vi "Update Outputs.vi"() -> ()   [LabVIEW 2012]
uses:
  <vilib>/Rock Robotics/WPI/Solenoid/WPI_SolenoidValue.ctl
  <vilib>/Rock Robotics/WPI/RobotDrive/WPI_RobotDriveGetSetRefNum.vi
  Robot Global Data.vi
  <vilib>/Rock Robotics/WPI/Solenoid/WPI_SolenoidSetEnum.vi
  <vilib>/Rock Robotics/WPI/RobotDrive/WPI_RobotDriveArcadeDrive_Standard(NoSaturation).vi
panel:
  out "Gyro Angle":dbl(knob) scale=0.0..360.0
  out "Loop Time 2":u32(graph)
  out "Right Distance (ft)":dbl
  out "Left Distance (ft)":dbl
  out "Right Rate":dbl(graph)
  out "Left Rate":dbl(graph)
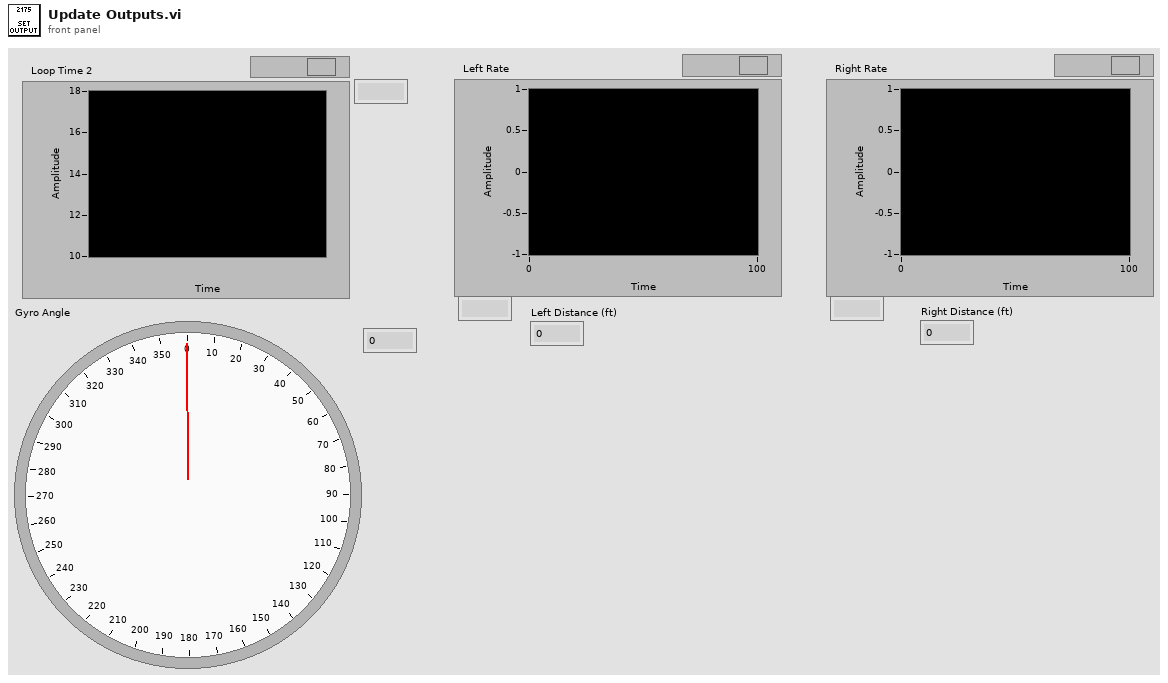
[diagram p1: front panel]
types:
  T1 = typedef "WPI_SolenoidDevRef.ctl" = cluster{"DevStatus":errorcluster, "Solenoid Module":T2, "Forward Solenoid Channel":T3, "Reverse Solenoid Channel":T3}
  T2 = typedef "FPGA_TypedefSolenoidModule.ctl" = enum16{"Solenoid Module 1", "Solenoid Module 2"}
  T3 = typedef "WPI_SolenoidChannel.ctl" = enum8{"Solenoid 1", "Solenoid 2", "Solenoid 3", "Solenoid 4", "Solenoid 5", "Solenoid 6", "Solenoid 7", "Solenoid 8", "Invalid"}
  T4 = typedef "WPI_RobotDriveDevRef.ctl" = cluster{"DevStatus":errorcluster, "Motors[]":T5[], "Square Inputs":bool, "Max Output":dbl, "Isochronous":bool}
  T5 = typedef "WPI_MotorControlDeviceRef.ctl" = cluster{"DeviceStatus":errorcluster, "Type":enum16{"PWM", "CAN"}, "PWM":cluster{"Digital Module":T6, "PWM Channel":T7, "DeadBand":T8}, "CAN":cluster{"Device Number":u8, "Control Mode":T9, "Semaphore":T10, "Max Vout":dbl}, "Invert":bool, "TransformRef":T11, "InvTransformRef":T11}
  T6 = typedef "FPGA_TypedefDigitalModule.ctl" = enum16{"Digital Module 1", "Digital Module 2"}
  T7 = typedef "FPGA_DIOPWMChannel.ctl" = enum8{"PWM 1", "PWM 2", "PWM 3", "PWM 4", "PWM 5", "PWM 6", "PWM 7", "PWM 8", "PWM 9", "PWM 10", "Invalid"}
  T8 = typedef "WPI_PWMDeadband.ctl" = cluster{"Name":string, "maxPositivePwm":i32, "minPositivePwm":i32, "centerPwm":i32, "maxNegativePwm":i32, "minNegativePwm":i32, "angularRange":u16}
  T9 = typedef "WPI_CANJaguar_ControlMode.ctl" = enum8{"Percent VBus", "Current", "Speed", "Position", "Voltage"}
  T10 = typedef "Semaphore RefNum" = refnum<k1>
  T11 = typedef "WPI_PWMTransform_ConPane.ctl" = refnum<vi>
  T12 = typedef "WPI_DigitalInputDevRef.ctl" = cluster{"DevStatus":errorcluster, "DIO Channel":T13, "Digital Module":T6}
  T13 = typedef "FPGA_DIOChannel.ctl" = enum8{"DIO 1", "DIO 2", "DIO 3", "DIO 4", "DIO 5", "DIO 6", "DIO 7", "DIO 8", "DIO 9", "DIO 10", "DIO 11", "DIO 12", "DIO 13", "DIO 14", "Invalid"}
  T14 = typedef "WPI_EncoderDevRef.ctl" = cluster{"DevStatus":errorcluster, "EncoderIndex":T15, "CounterIndex":T16, "DistancePerCount":dbl, "Decoding Type":T17}
  T15 = typedef "FPGA_EncoderIdx.ctl" = enum8{"Enc 0", "Enc 1", "Enc 2", "Enc 3", "Invalid"}
  T16 = typedef "FPGA_CounterCtrSystemIndex.ctl" = enum8{"Ctr 0", "Ctr 1", "Ctr 2", "Ctr 3", "Ctr 4", "Ctr 5", "Ctr 6", "Ctr 7", "Invalid"}
  T17 = typedef "WPI_EncoderType.ctl" = enum16{"1x", "2x", "4x"}
  T18 = typedef "WPI_SolenoidValue.ctl" = enum16{"Off", "On", "Forward", "Reverse"}
  T19 = typedef "WPI_GyroDevRef.ctl" = cluster{"DevStatus":errorcluster, "Analog Module":T20, "Analog Channel":T21, "Offset":dbl, "Gain (VoltsPerDegree/Second)":dbl}
  T20 = typedef "FPGA_TypedefAnalogModule.ctl" = enum16{"Analog Module 1", "Analog Module 2"}
  T21 = typedef "FPGA_AIChannel.ctl" = enum8{"AI 1", "AI 2", "AI 3", "AI 4", "AI 5", "AI 6", "AI 7", "AI 8", "Invalid"}
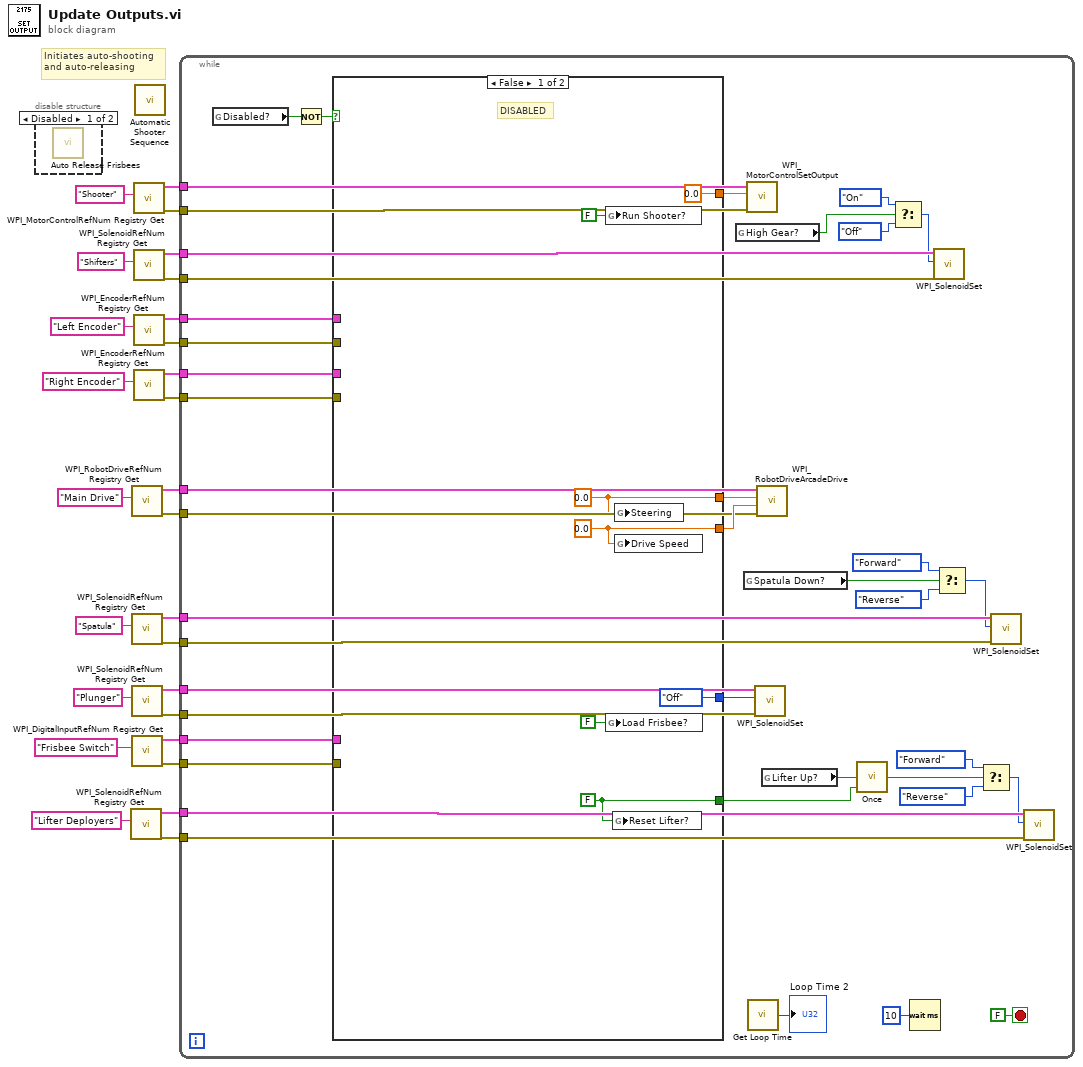
[diagram p0: block diagram]
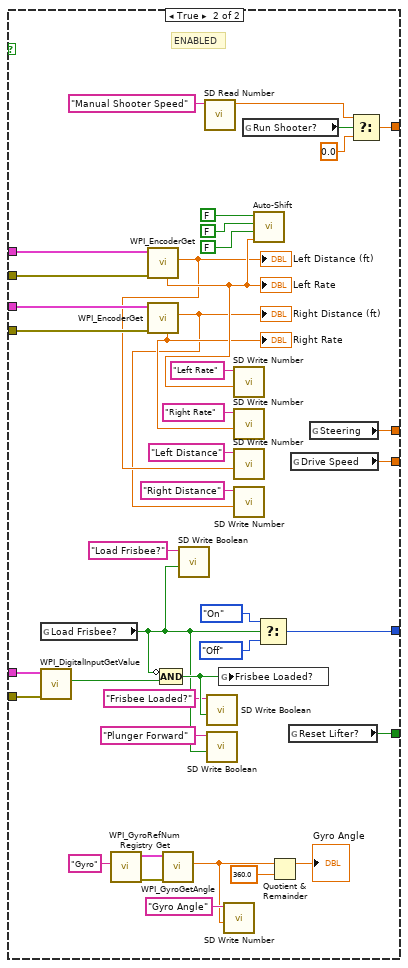
[diagram p3: hidden frame]
diagram:
  # "Initiates auto-shooting\nand auto-releasing"
  n1 = disable-structure shown="Disabled" {
    frame Disabled {
      n2 = call "Auto Release Frisbees.vi"() -> ()  [unwired: 12 in]
    }
    frame Enabled {
    }
  }
  n3 = call <vilib>:"WPI_SolenoidRefNum Registry Get.vi"("refnum name"="Lifter Deployers") -> ("error out"=w1:errorcluster, "SolenoidDevRef"=w2:T1)  [unwired: 9 in]
  n4 = call <vilib>:"WPI_RobotDriveRefNum Registry Get.vi"("refnum name"="Main Drive") -> ("error out"=w22:errorcluster, "RobotDriveDevRef"=w23:T4)  [unwired: 9 in]
  n5 = call <vilib>:"WPI_SolenoidRefNum Registry Get.vi"("refnum name"="Spatula") -> ("error out"=w16:errorcluster, "SolenoidDevRef"=w17:T1)  [unwired: 9 in]
  n6 = call <vilib>:"WPI_SolenoidRefNum Registry Get.vi"("refnum name"="Plunger") -> ("error out"=w15:errorcluster, "SolenoidDevRef"=w14:T1)  [unwired: 9 in]
  n7 = call <vilib>:"WPI_DigitalInputRefNum Registry Get.vi"("refnum name"="Frisbee Switch") -> ("error out"=w4:errorcluster, "DigitalInputDevRef"=w5:T12)  [unwired: 9 in]
  n8 = call <vilib>:"WPI_MotorControlRefNum Registry Get.vi"("refnum name"="Shooter") -> ("error out"=w25:errorcluster, "MotorControlDevRef"=w26:T5)  [unwired: 9 in]
  n9 = call <vilib>:"WPI_SolenoidRefNum Registry Get.vi"("refnum name"="Shifters") -> ("error out"=w19:errorcluster, "SolenoidDevRef"=w20:T1)  [unwired: 9 in]
  n10 = call <vilib>:"WPI_EncoderRefNum Registry Get.vi"("refnum name"="Left Encoder") -> ("error out"=w10:errorcluster, "EncoderDevRef"=w11:T14)  [unwired: 9 in]
  n11 = call <vilib>:"WPI_EncoderRefNum Registry Get.vi"("refnum name"="Right Encoder") -> ("error out"=w9:errorcluster, "EncoderDevRef"=w8:T14)  [unwired: 9 in]
  n12 = call "Automatic Shooter Sequence.vi"() -> ()  [unwired: 12 in]
  n13 = while {
    tunnel: w26 -> [w64]
    tunnel: w25 -> [w63]
    tunnel: w23 -> [w60]
    tunnel: w22 -> [w59]
    tunnel: w20 -> [w58]
    tunnel: w19 -> [w57]
    tunnel: w17 -> [w55]
    tunnel: w16 -> [w56]
    tunnel: w14 -> [w54]
    tunnel: w15 -> [w53]
    tunnel: w11 -> [w50]
    tunnel: w10 -> [w49]
    tunnel: w8 -> [w47]
    tunnel: w9 -> [w48]
    tunnel: w5 -> [w46]
    tunnel: w4 -> [w45]
    tunnel: w2 -> [w44]
    tunnel: w1 -> [w43]
    stop <- FALSE stop-if-true
    n14 = global read "Robot Global Data.vi" "Disabled?"() -> (w66:bool)
    n15 = Not(x=w66) -> (.not. x?=w65:bool)
    n16 = case shown="False" w65 {
      tunnel: [0.0 ("Output") w104] -> w51
      tunnel: [w69 w116] -> w62
      tunnel: [w70 w109] -> w61
      tunnel: [WPI_SolenoidValue."Off" ("Value") w111] -> w52
      tunnel: w50 -> [_ w108]
      tunnel: w49 -> [_ w107]
      tunnel: w47 -> [_ w101]
      tunnel: w48 -> [_ w102]
      tunnel: w46 -> [_ w100]
      tunnel: w45 -> [_ w99]
      tunnel: [w71 w95] -> w36
      frame False {
        w71 = FALSE ("High Gear?")
        w70 = 0.0 ("Drive Speed")
        w69 = 0.0 ("Steering")
        # "DISABLED"
        n17 = global write "Robot Global Data.vi" "Run Shooter?"(FALSE ("High Gear?")) -> ()
        n18 = global write "Robot Global Data.vi" "Load Frisbee?"(FALSE ("High Gear?")) -> ()
        n19 = global write "Robot Global Data.vi" "Reset Lifter?"(w71) -> ()
        n20 = global write "Robot Global Data.vi" "Steering"(w69) -> ()
        n21 = global write "Robot Global Data.vi" "Drive Speed"(w70) -> ()
      }
      frame True {
        # "ENABLED"
        n22 = global read "Robot Global Data.vi" "Load Frisbee?"() -> (w91:bool)
        n23 = call <vilib>:"WPI_DigitalInputGetValue.vi"("error in (no error)"=w99, "DigitalInputDevRef"=w100) -> ("Value"=w98:bool)  [unwired: 7 in, 2 out]
        n24 = call <vilib>:"WPI_GyroRefNum Registry Get.vi"("refnum name"="Gyro") -> ("error out"=w81:errorcluster, "GyroDevRef"=w80:T19)  [unwired: 9 in]
        n25 = call <vilib>:"WPI_EncoderGet.vi"("error in (no error)"=w107, "EncoderDevRef"=w108) -> ("Distance"=w84:dbl, "Rate"=w86:dbl)  [unwired: 4 in, 4 out]
        "Left Rate" <- w86
        "Left Distance (ft)" <- w84
        n26 = call <vilib>:"WPI_EncoderGet.vi"("error in (no error)"=w102, "EncoderDevRef"=w101) -> ("Distance"=w83:dbl, "Rate"=w85:dbl)  [unwired: 4 in, 4 out]
        "Right Rate" <- w85
        "Right Distance (ft)" <- w83
        n27 = Compound Arithmetic op=AND(invert w91, w98) -> (w97:bool)
        n28 = call <vilib>:"WPI_GyroGetAngle.vi"("error in (no error)"=w81, "GyroDevRef"=w80) -> ("Angle"=w78:dbl)  [unwired: 6 in, 3 out]
        n29 = call <vilib>:"SD Write Boolean.vi"("Boolean"=w91, "Name"="Load Frisbee?") -> ()  [unwired: 8 in, 2 out]
        n30 = call <vilib>:"SD Read Number.vi"("Name"="Manual Shooter Speed") -> ("Numeric"=w105:dbl)  [unwired: 8 in, 2 out]
        n31 = call <vilib>:"SD Write Boolean.vi"("Boolean"=w97, "Name"="Frisbee Loaded?") -> ()  [unwired: 8 in, 2 out]
        n32 = call <vilib>:"SD Write Boolean.vi"("Boolean"=w91, "Name"="Plunger Forward") -> ()  [unwired: 8 in, 2 out]
        n33 = global write "Robot Global Data.vi" "Frisbee Loaded?"(w97) -> ()
        n34 = call <vilib>:"SD Write Number.vi"("Numeric"=w78, "Name"="Gyro Angle") -> ()  [unwired: 8 in, 2 out]
        n35 = call <vilib>:"SD Write Number.vi"("Numeric"=w86, "Name"="Left Rate") -> ()  [unwired: 8 in, 2 out]
        n36 = call <vilib>:"SD Write Number.vi"("Numeric"=w85, "Name"="Right Rate") -> ()  [unwired: 8 in, 2 out]
        n37 = call <vilib>:"SD Write Number.vi"("Numeric"=w84, "Name"="Left Distance") -> ()  [unwired: 8 in, 2 out]
        n38 = call <vilib>:"SD Write Number.vi"("Numeric"=w83, "Name"="Right Distance") -> ()  [unwired: 8 in, 2 out]
        n39 = global read "Robot Global Data.vi" "Run Shooter?"() -> (w106:bool)
        n40 = call "Auto-Shift.vi"("Average Ft/Sec"=w86, "Coastdown Enabled?"=FALSE, "Kickdown Enabled?"=FALSE, "Upshift Enabled?"=FALSE) -> ()  [unwired: 1 in]
        n41 = Select(t=WPI_SolenoidValue."On" ("Value"), s=w91, f=WPI_SolenoidValue."Off" ("Value")) -> (s? t:f=w111:T18)
        n42 = Quotient & Remainder(x=w78, y=360.0) -> (x-y*floor(x/y)=→"Gyro Angle":dbl)  [unwired: 1 out]
        n43 = global read "Robot Global Data.vi" "Reset Lifter?"() -> (w95:bool)
        n44 = global read "Robot Global Data.vi" "Drive Speed"() -> (w109:dbl)
        n45 = global read "Robot Global Data.vi" "Steering"() -> (w116:dbl)
        n46 = Select(t=w105, s=w106, f=0.0) -> (s? t:f=w104:dbl)
      }
    }
    n47 = global read "Robot Global Data.vi" "High Gear?"() -> (w29:bool)
    n48 = global read "Robot Global Data.vi" "Spatula Down?"() -> (w35:bool)
    n49 = call <vilib>:"WPI_MotorControlSetOutput.vi"("error in (no error)"=w63, "Output"=w51, "MotorControlDevRef"=w64) -> ()  [unwired: 6 in, 3 out]
    n50 = call "Get Loop Time.vi"() -> ("Loop Time"=→"Loop Time 2":u32)  [unwired: 1 in]
    n51 = call-poly <vilib>:"WPI_SolenoidSet.vi"("error in (no error)"=w53, "Value"=w52, "SolenoidDevRef"=w54) -> ()  [unwired: 7 in, 2 out]
    n52 = call-poly <vilib>:"WPI_RobotDriveArcadeDrive.vi"("error in (no error)"=w59, "Y axis value"=w61, "X axis value"=w62, "RobotDriveDevRef"=w60) -> ()  [unwired: 5 in, 3 out]
    n53 = global read "Robot Global Data.vi" "Lifter Up?"() -> (w38:bool)
    n54 = call "Once.vi"("Reset?"=w36, "Input"=w38) -> ("Output"=w37:bool)  [unwired: 1 in]
    n55 = Select(t=WPI_SolenoidValue."On" ("Value"), s=w29, f=WPI_SolenoidValue."Off" ("Value")) -> (s? t:f=w28:T18)
    n56 = Wait (ms)(milliseconds to wait=u32 10) -> ()  [unwired: 1 out]
    n57 = call-poly <vilib>:"WPI_SolenoidSet.vi"("error in (no error)"=w57, "Value"=w28, "SolenoidDevRef"=w58) -> ()  [unwired: 7 in, 2 out]
    n58 = Select(t=WPI_SolenoidValue."Forward" ("Value"), s=w35, f=WPI_SolenoidValue."Reverse" ("Value")) -> (s? t:f=w32:T18)
    n59 = Select(t=WPI_SolenoidValue."Forward" ("Value"), s=w37, f=WPI_SolenoidValue."Reverse" ("Value")) -> (s? t:f=w39:T18)
    n60 = call-poly <vilib>:"WPI_SolenoidSet.vi"("error in (no error)"=w56, "Value"=w32, "SolenoidDevRef"=w55) -> ()  [unwired: 7 in, 2 out]
    n61 = call-poly <vilib>:"WPI_SolenoidSet.vi"("error in (no error)"=w43, "Value"=w39, "SolenoidDevRef"=w44) -> ()  [unwired: 7 in, 2 out]
  }
